vi "Create Analog Replay.vi"(8 "error in (no error)":errorcluster, 9 "Analog Replay Data Options":T1={"Input file"=path "", "Group"="", "Channel"="", "Reverse"=FALSE, "FPGA Memory Size"=enum."16,384", "Position reference"=enum."Crank angle", "Data selection method"=enum."Manual", "Offset"=0, "Samples"=0, "Missing teeth location"=0.0, "DataPlugin"=""}, 10 "Analog Replay Settings":T5={"Name"="", "Name in bitfile"="", "DAC bipolar range (V)"=0.0, "Voltage below min speed"=0.0, "Min speed (RPM)"=0.0, "Voltage at min speed"=0.0, "Max speed (RPM)"=0.0, "Voltage at max speed"=0.0, "Negate playback voltage values at negative engine speed"=TRUE, "Allow run-time override of voltage scaling"=FALSE}, 11 "APU Node in":refnum<k24>) -> (0 "error out":errorcluster, 3 "APU Node out":refnum<k24>)   [LabVIEW 2015, in "Engine Simulation Toolkit SysDef API.lvlib"]
uses:
  Engine Simulation Toolkit SysDef API.lvlib
  Analog Replay Settings.ctl
  NationalInstruments.VeriStand.SystemDefinitionAPI
  Analog Replay Data Options.ctl
  System Explorer/FPGA Mem Size.ctl
  System Explorer/Position Reference.ctl
  System Explorer/Data Replay Data Selection Method.ctl
  System Explorer/File Load Dialog.ctl
  <vilib>/Platform/storage/utility/usiPluginInformation.ctl
  <vilib>/NI Veristand/Custom Device API/Custom Device Channel Type.ctl
  Shared/Constants and GUIDs.vi
  Shared/Properties.vi
  <vilib>/NI/NI VeriStand Advanced SysDef API/_SubVIs/SysDef.Property.Set.DBL.vi
  <vilib>/NI/NI VeriStand Advanced SysDef API/_SubVIs/SysDef.Property.Set.Boolean.vi
  System Explorer/Engine Simulation Toolkit System Explorer.lvlib
  Shared/Engine Simulation Toolkit Shared.lvlib
  <vilib>/NI Veristand/Custom Device API/Custom Device API.lvlib
  <vilib>/NI/NI VeriStand Advanced SysDef API/SysDef API/Advanced System Definition.lvlib
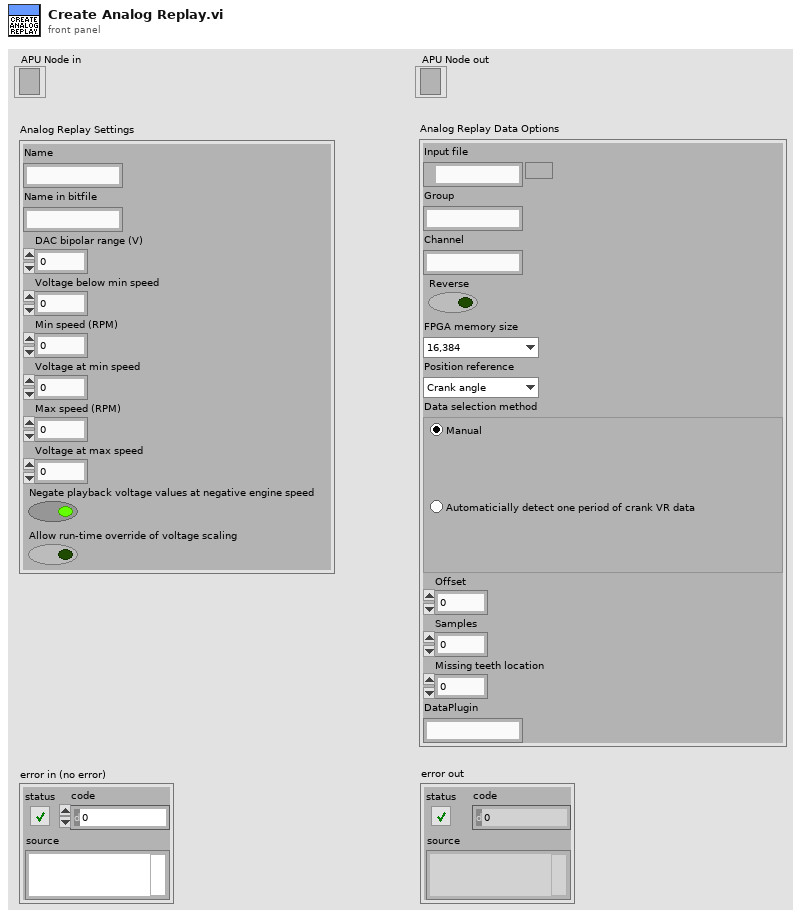
[diagram p1: front panel]
types:
  T1 = typedef "Engine Simulation Toolkit SysDef API.lvlib/Analog Replay Data Options.ctl" = cluster{"Input file":path, "Group":string, "Channel":string, "Reverse":bool, "FPGA Memory Size":T2, "Position reference":T3, "Data selection method":T4, "Offset":i32, "Samples":i32, "Missing teeth location":dbl, "DataPlugin":string}
  T2 = typedef "Engine Simulation Toolkit System Explorer.lvlib/FPGA Mem Size.ctl" = enum16{"65,536", "32,768", "16,384", "8,192", "4,096", "2,048", "1,024"}
  T3 = typedef "Engine Simulation Toolkit System Explorer.lvlib/Position Reference.ctl" = enum16{"Crank angle", "Cycle angle"}
  T4 = typedef "Engine Simulation Toolkit System Explorer.lvlib/Data Replay Data Selection Method.ctl" = enum32{"Manual", "AutoVRCrank"}
  T5 = typedef "Engine Simulation Toolkit SysDef API.lvlib/Analog Replay Settings.ctl" = cluster{"Name":string, "Name in bitfile":string, "DAC bipolar range (V)":dbl, "Voltage below min speed":dbl, "Min speed (RPM)":dbl, "Voltage at min speed":dbl, "Max speed (RPM)":dbl, "Voltage at max speed":dbl, "Negate playback voltage values at negative engine speed":bool, "Allow run-time override of voltage scaling":bool}
  T6 = typedef "Engine Simulation Toolkit System Explorer.lvlib/File Load Dialog.ctl" = cluster{"File":path, "Group":string, "Channel":string, "DataPlugin":string, "MissingTeeth":dbl, "ErrState":string, "File Selected":bool, "Data Selection Method":T4, "Offset":i32, "Length":i32, "DataPlugins Info":T7[], "Controls":refnum<vi>[], "File Ref":refnum<k20>, "Groups":string[], "Channels":string[], "Groups Refs":refnum<k20>[], "Channel Refs":refnum<k20>[], "Cancelled":bool, "Position reference":T3, "FPGA memory size":T2, "GroupRef":refnum<k20>, "ChanRef":refnum<k20>, "Data":dbl[], "ReverseData":bool, "DispTwoRotations":bool, "cycle range":u16}
  T7 = typedef "usiPluginInformation.ctl" = cluster{"name":string, "version":string, "type":string, "read-only?":bool, "extensions":string[]}
  T8 = typedef "Custom Device API.lvlib/Custom Device Channel Type.ctl" = enum16{"Input", "Output"}
  T9 = typedef "Custom Device API.lvlib/Custom Device Item Ref.ctl" = u64
  T10 = typedef "Engine Simulation Toolkit Shared.lvlib/Channel.ctl" = cluster{"Name":string, "Units":string, "Default":dbl, "Description":string, "Scalable":bool}
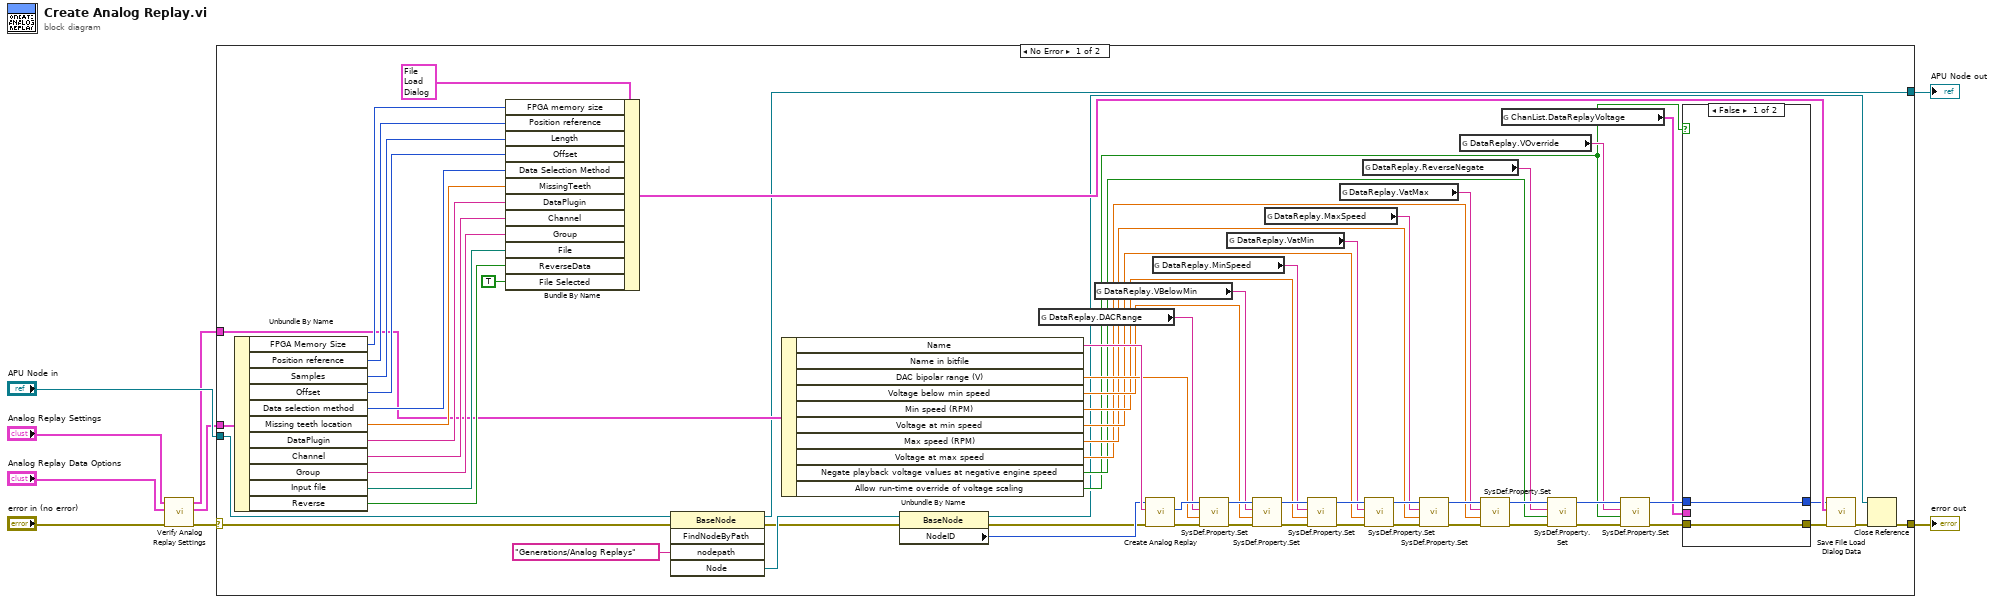
[diagram p0: block diagram]
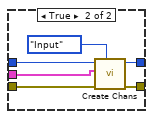
[diagram p2: hidden frame]
diagram:
  n1 = call "Verify Analog Replay Settings.vi"("error in (no error)"="error in (no error)", "Analog Replay Data Options in"="Analog Replay Data Options", "Analog Replay Settings in"="Analog Replay Settings") -> ("error out"=w5:errorcluster, "Analog Replay Data Options out"=w1:T1, "Analog Replay Settings out"=w3:T5)  [unwired: 6 in]
  n2 = case shown="No Error" w5 {
    selector: w5 -> [w16 w84]
    tunnel: "APU Node in" -> [w18 w83]
    tunnel: [w14 w83] -> w8
    tunnel: [w12 w84] -> w7
    tunnel: w3 -> [w20 _]
    tunnel: w1 -> [w19 _]
    frame No Error {
      n3 = Unbundle By Name(w19) -> ("FPGA Memory Size"=w64:T2, "Position reference"=w65:T3, "Samples"=w22:i32, "Offset"=w23:i32, "Data selection method"=w25:T4, "Missing teeth location"=w24:dbl, "DataPlugin"=w21:string, "Channel"=w66:string, "Group"=w67:string, "Input file"=w68:path, "Reverse"=w69:bool)
      n4 = Bundle By Name(cluster=T6 {"File"=path "", "Group"="", "Channel"="", "DataPlugin"="", "MissingTeeth"=0.0, "ErrState"="", "File Selected"=FALSE, "Data Selection Method"=enum."Manual", "Offset"=0, "Length"=0, "DataPlugins Info"=[], "Controls"=[], "File Ref"=refnum, "Groups"=[], "Channels"=[], "Groups Refs"=[], "Channel Refs"=[], "Cancelled"=FALSE, "Position reference"=enum."Crank angle", "FPGA memory size"=enum."32,768", "GroupRef"=refnum, "ChanRef"=refnum, "Data"=[], "ReverseData"=FALSE, "DispTwoRotations"=FALSE, "cycle range"=720} ("FileDialog"), "FPGA memory size"=w64, "Position reference"=w65, "Length"=w22, "Offset"=w23, "Data Selection Method"=w25, "MissingTeeth"=w24, "DataPlugin"=w21, "Channel"=w66, "Group"=w67, "File"=w68, "ReverseData"=w69, "File Selected"=TRUE) -> (w70:T6)
      n5 = invoke class="BaseNode" method="FindNodeByPath"(reference=w18, error in=w16, "nodepath"="Generations/Analog Replays") -> (reference out=w14:refnum<k24>, error out=w15:errorcluster, "Node"=w17:refnum<k24>)  [unwired: 2 in, 2 out]
      n6 = Unbundle By Name(w20) -> ("Name"=w74:string, "DAC bipolar range (V)"=w59:dbl, "Voltage below min speed"=w56:dbl, "Min speed (RPM)"=w48:dbl, "Voltage at min speed"=w46:dbl, "Max speed (RPM)"=w45:dbl, "Voltage at max speed"=w42:dbl, "Negate playback voltage values at negative engine speed"=w33:bool, "Allow run-time override of voltage scaling"=w31:bool)  [unwired: 1 out]
      n7 = property class="BaseNode"(reference=w17, error in=w15) -> (reference out=w11:refnum<k24>, error out=w72:errorcluster, "NodeID"=w73:u64)
      n8 = global read "Properties.vi" "DataReplay.DACRange"() -> (w60:string)
      n9 = global read "Properties.vi" "DataReplay.VBelowMin"() -> (w55:string)
      n10 = call "Create Analog Replay.vi"("error in (no error)"=w72, "analog replay name"=w74, "Section Ptr"=w73) -> ("error out"=w61:errorcluster, "Analog replay ref"=w62:T9)  [unwired: 6 in, 1 out]
      n11 = global read "Properties.vi" "DataReplay.MinSpeed"() -> (w47:string)
      n12 = call-poly <vilib>:"SysDef.Property.Set.vi"("error in (no error)"=w61, "Value"=w59, "Property Name"=w60, "nodeID"=w62) -> ("error out"=w57:errorcluster, "nodeID out"=w58:u64)  [unwired: 6 in]
      n13 = global read "Properties.vi" "DataReplay.VatMin"() -> (w41:string)
      n14 = call-poly <vilib>:"SysDef.Property.Set.vi"("error in (no error)"=w57, "Value"=w56, "Property Name"=w55, "nodeID"=w58) -> ("error out"=w49:errorcluster, "nodeID out"=w50:u64)  [unwired: 6 in]
      n15 = global read "Properties.vi" "DataReplay.MaxSpeed"() -> (w40:string)
      n16 = call-poly <vilib>:"SysDef.Property.Set.vi"("error in (no error)"=w49, "Value"=w48, "Property Name"=w47, "nodeID"=w50) -> ("error out"=w54:errorcluster, "nodeID out"=w53:u64)  [unwired: 6 in]
      n17 = global read "Properties.vi" "DataReplay.VatMax"() -> (w39:string)
      n18 = global read "Properties.vi" "DataReplay.ReverseNegate"() -> (w34:string)
      n19 = call-poly <vilib>:"SysDef.Property.Set.vi"("error in (no error)"=w54, "Value"=w46, "Property Name"=w41, "nodeID"=w53) -> ("error out"=w52:errorcluster, "nodeID out"=w51:u64)  [unwired: 6 in]
      n20 = call-poly <vilib>:"SysDef.Property.Set.vi"("error in (no error)"=w52, "Value"=w45, "Property Name"=w40, "nodeID"=w51) -> ("error out"=w44:errorcluster, "nodeID out"=w43:u64)  [unwired: 6 in]
      n21 = global read "Properties.vi" "DataReplay.VOverride"() -> (w32:string)
      n22 = call-poly <vilib>:"SysDef.Property.Set.vi"("error in (no error)"=w44, "Value"=w42, "Property Name"=w39, "nodeID"=w43) -> ("error out"=w38:errorcluster, "nodeID out"=w37:u64)  [unwired: 6 in]
      n23 = global read "Constants and GUIDs.vi" "ChanList.DataReplayVoltage"() -> (w26:T10[])
      n24 = call-poly <vilib>:"SysDef.Property.Set.vi"("error in (no error)"=w38, "Value"=w33, "Property Name"=w34, "nodeID"=w37) -> ("error out"=w36:errorcluster, "nodeID out"=w35:u64)  [unwired: 6 in]
      n25 = call-poly <vilib>:"SysDef.Property.Set.vi"("error in (no error)"=w36, "Value"=w31, "Property Name"=w32, "nodeID"=w35) -> ("error out"=w30:errorcluster, "nodeID out"=w29:u64)  [unwired: 6 in]
      n26 = case shown="False" w31 {
        tunnel: w30 -> [w76 w80]
        tunnel: w29 -> [w75 w81]
        tunnel: [w76 w79] -> w28
        tunnel: [w75 w78] -> w27
        tunnel: w26 -> [_ w77]
        frame False {
        }
        frame True {
          n27 = call "Create Chans.vi"("Type"=Custom_Device_Channel_Type."Input", "error in (no error)"=w80, "Channels"=w77, "Section Ptr"=w81) -> ("error out"=w79:errorcluster, "Section Ptr dup"=w78:T9)  [unwired: 4 in, 2 out]
        }
      }
      n28 = call "Save File Load Dialog Data.vi"("error in (no error)"=w28, "FileDialog"=w70, "Node Ptr"=w27) -> ("error out"=w13:errorcluster)  [unwired: 8 in]
      n29 = Close Reference(reference=w11, error in (no error)=w13) -> (error out=w12:errorcluster)
    }
    frame Error {
    }
  }
  "APU Node out" <- w8
  "error out" <- w7
